vi "上转向轴压装.vi"() -> ()   [LabVIEW 2020]
uses:
  Global_Variable/Global.vi
  Global_Variable/A131258.vi
  Database/Global1.vi
  <vilib>/addons/database/Connection.llb/DB Tools Open Connec (String).vi
  <vilib>/addons/database/Connection.llb/Conn Execute.vi
  <vilib>/addons/database/Recordset.llb/Rec Fetch Recordset Data (R).vi
  <vilib>/addons/database/NI_Database_API.lvlib
panel:
  out "标尺_Event":refnum<user-event>
  out "压装曲线":cluster{dbl[], dbl[]}[](graph)
  out "RESULT":string
  out "PRODUCTID":string
  out "USERID":string
  out "前序deviceID":string
  out "deviceID":string
  out "CODE_ID":string
  in  "判定结果 3":bool[][](array[boolean])=[[TRUE]]
  out "第一段压装位移内波动压力(KN)":dbl format="%_5g"
  out "第二段压装位移内波动压力(KN)":dbl format="%_5g"
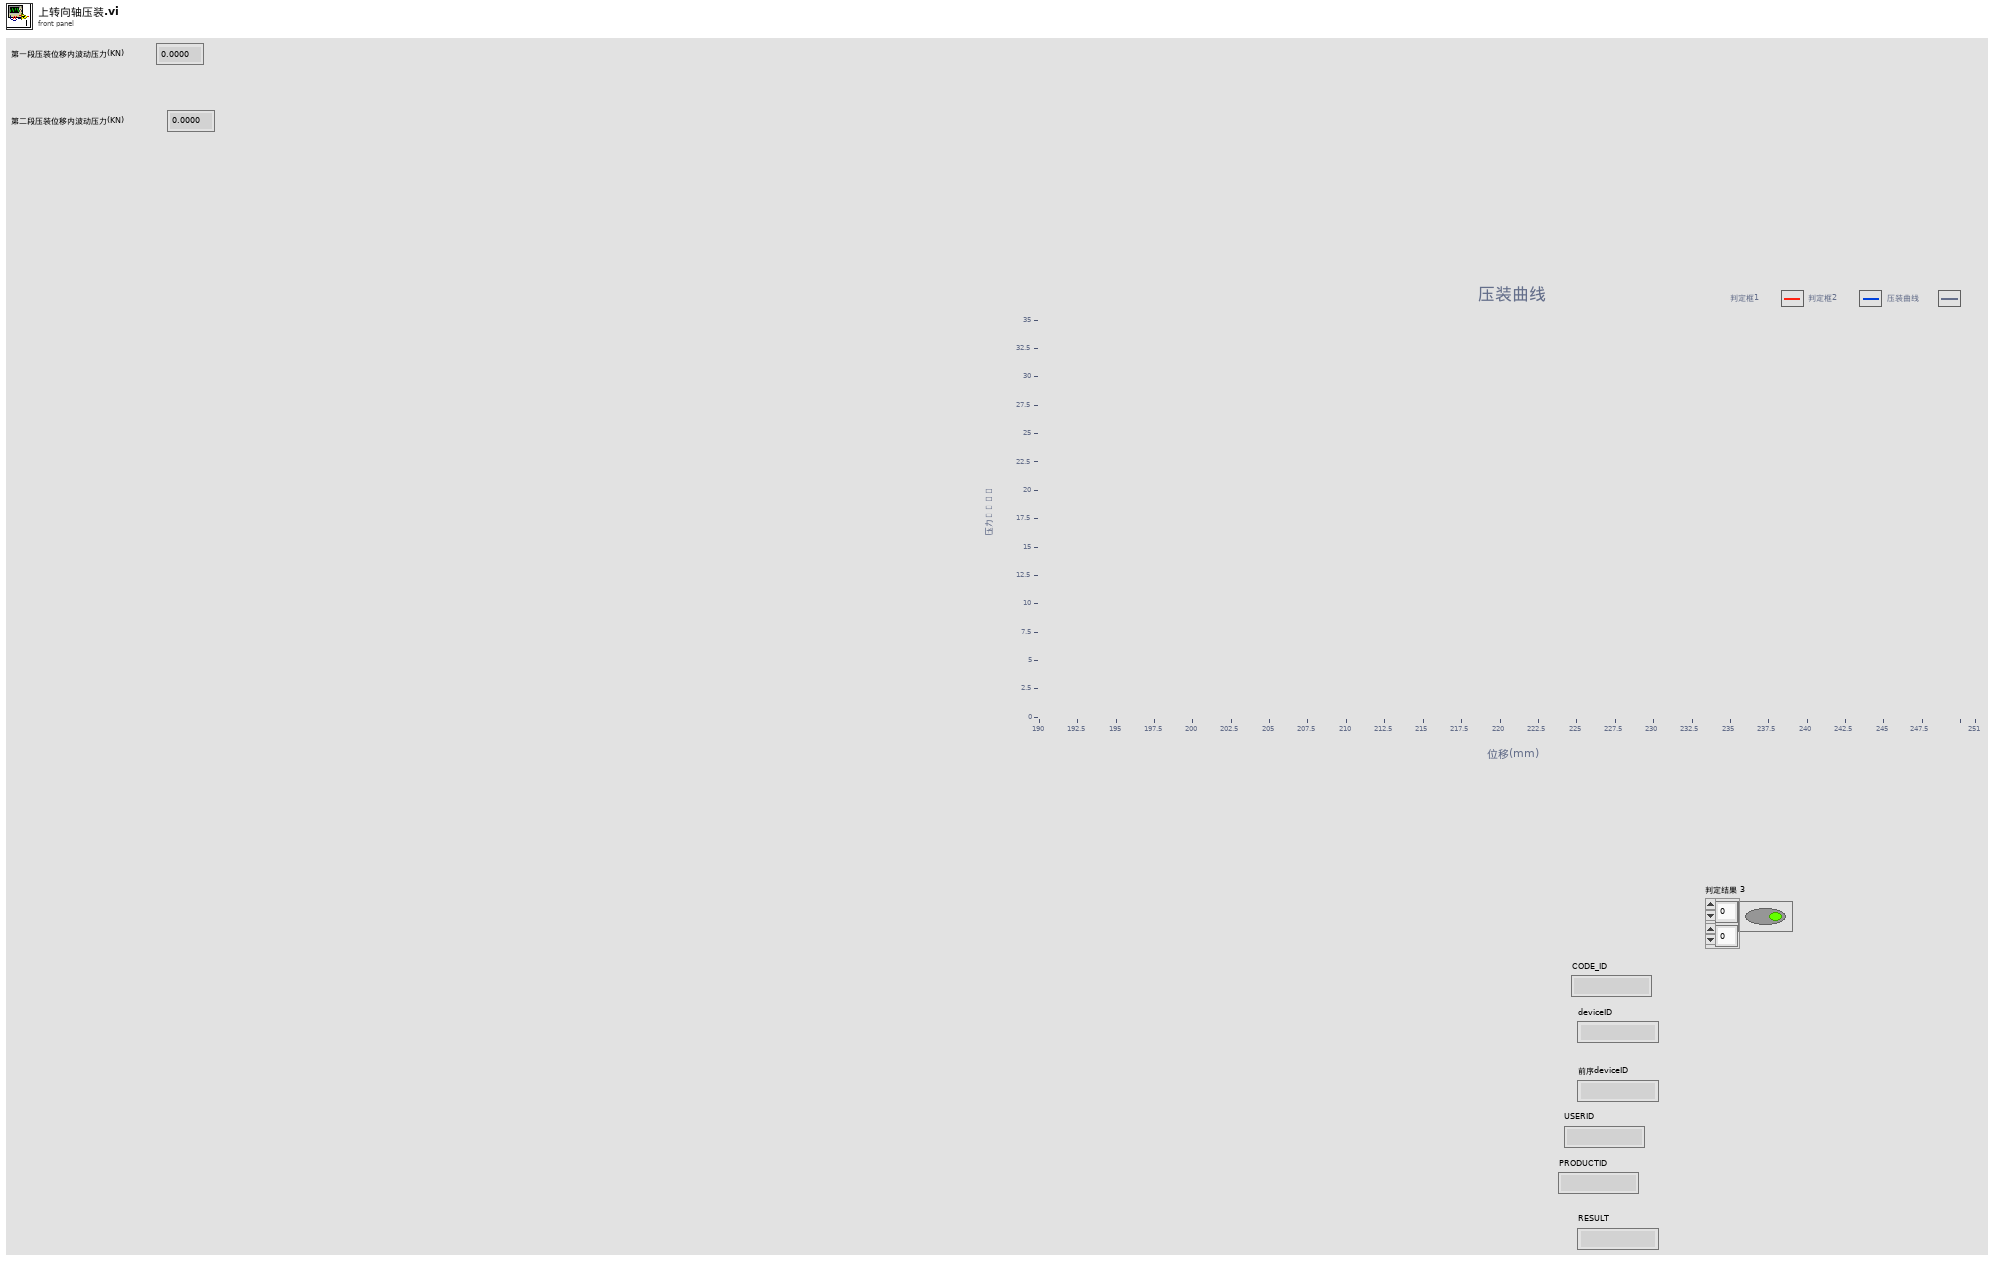
[diagram p1: front panel]
types:
  T1 = cluster{"第一段判定框位移":cluster{"单位":string, "下限":dbl, "上限":dbl}, "第一段判定框压力":cluster{"单位":string, "下限":dbl, "上限":dbl}, "低二段判定框位移":cluster{"单位":string, "下限":dbl, "上限":dbl}, "第二段判定框压力":cluster{"单位":string, "下限":dbl, "上限":dbl}}
  T2 = cluster{"第一段压力最大值":cluster{"单位":string, "下限":dbl, "上限":dbl}, "第一段压力最小值":cluster{"单位":string, "下限":dbl, "上限":dbl}, "压装最终位移":cluster{"单位":string, "下限":dbl, "上限":dbl}}
  T3 = cluster{"第一段压力最大值":cluster{"单位":string, "下限":dbl, "上限":dbl}, "第一段压力最小值":cluster{"单位":string, "下限":dbl, "上限":dbl}, "第二段压力最大值":cluster{"单位":string, "下限":dbl, "上限":dbl}, "第二段压力最小值":cluster{"单位":string, "下限":dbl, "上限":dbl}, "压装最终位移":cluster{"单位":string, "下限":dbl, "上限":dbl}}
  T4 = typedef "NI_Database_API.lvlib/Conn ObjectReference.ctl" = refnum<k1>
  T5 = typedef "NI_Database_API.lvlib/Rec ObjectReference.ctl" = refnum<k1>
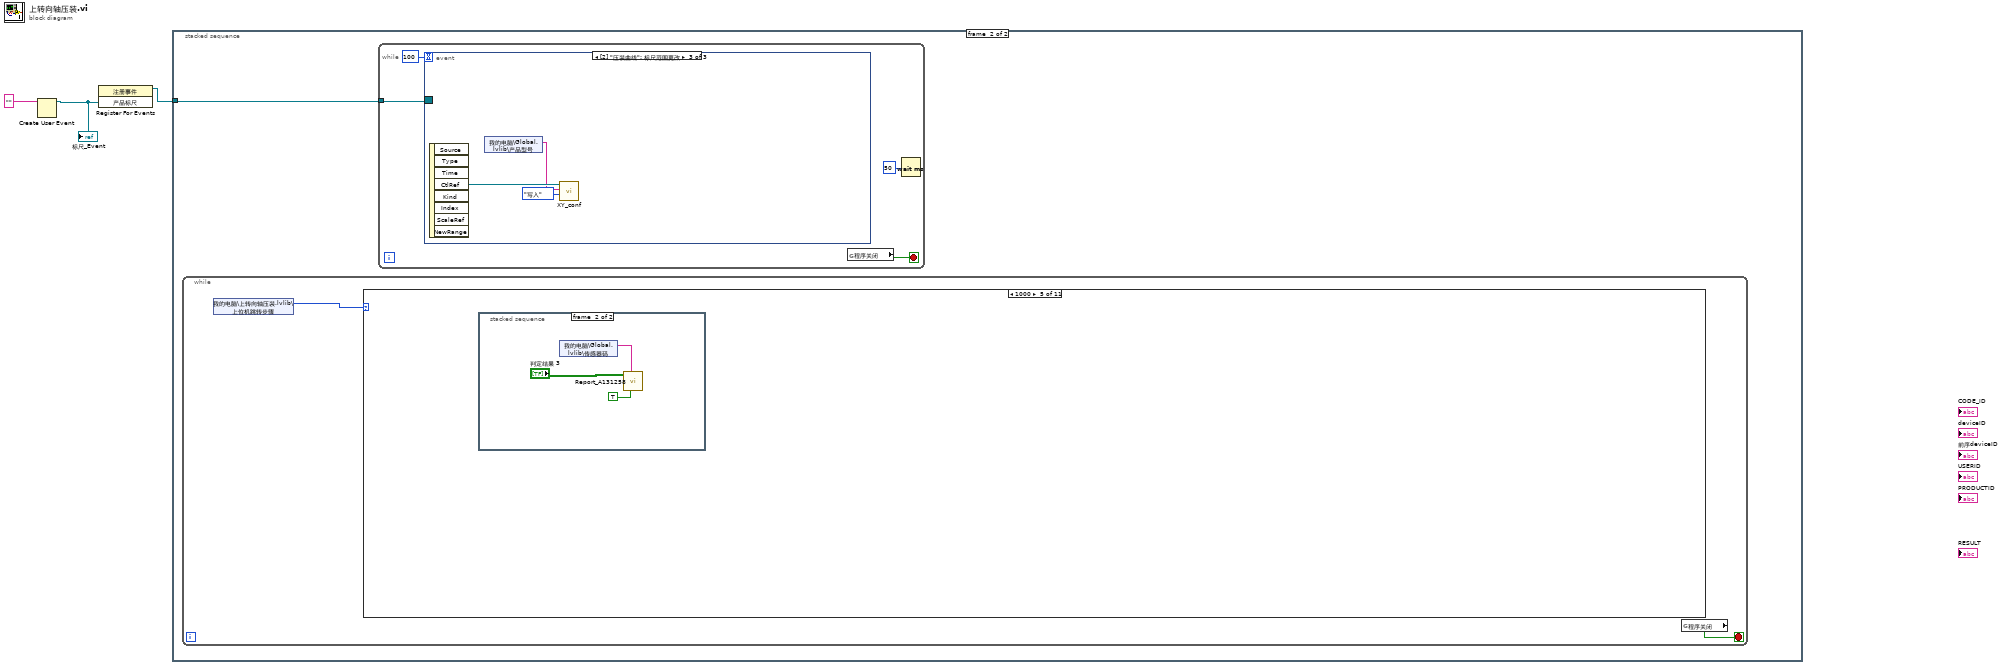
[diagram p0: block diagram]
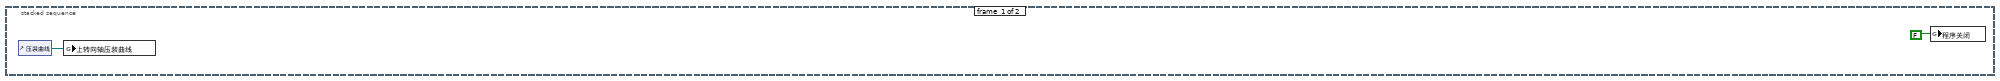
[diagram p2: hidden frame]
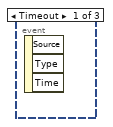
[diagram p3: hidden frame]
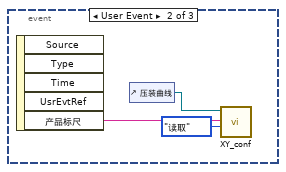
[diagram p4: hidden frame]
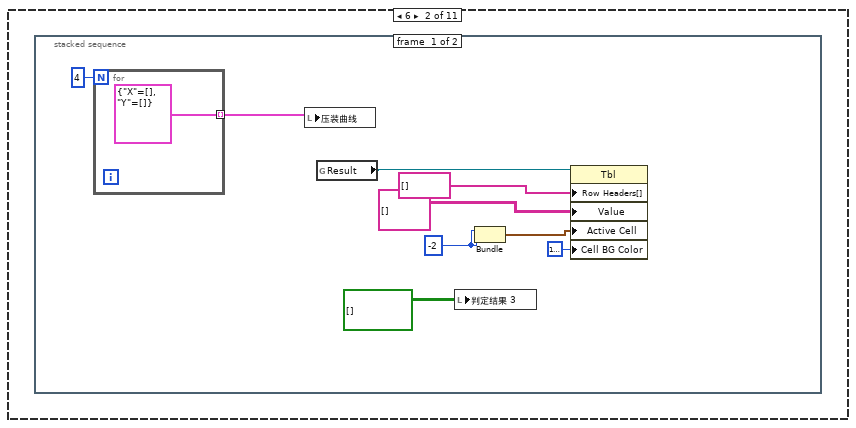
[diagram p6: hidden frame]
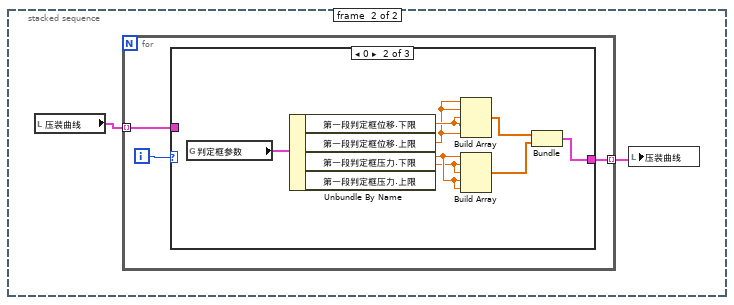
[diagram p7: hidden frame]
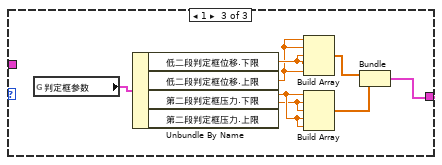
[diagram p9: hidden frame]
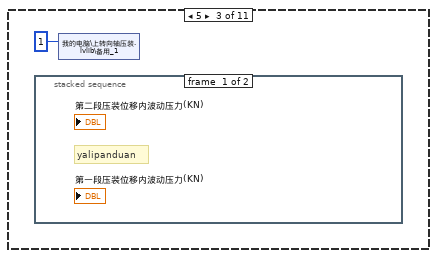
[diagram p10: hidden frame]
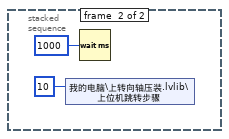
[diagram p11: hidden frame]
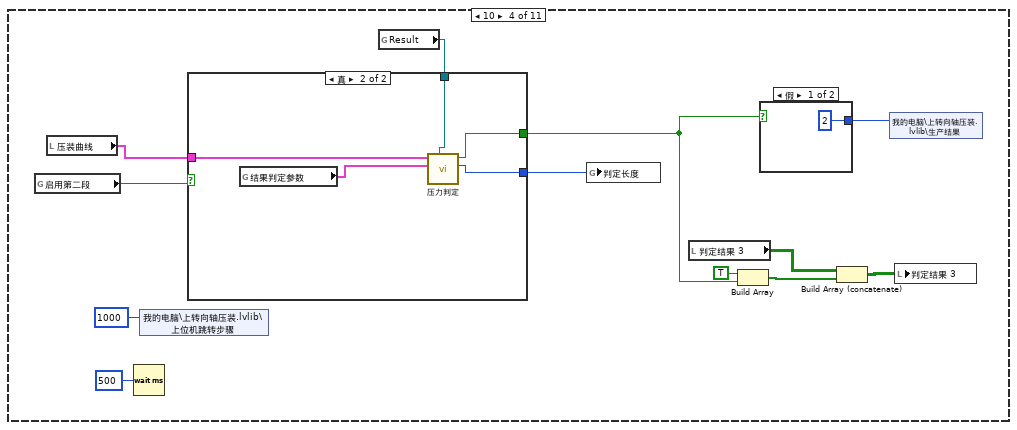
[diagram p12: hidden frame]
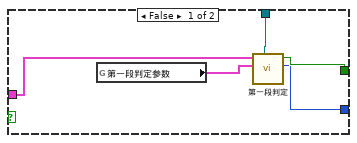
[diagram p13: hidden frame]
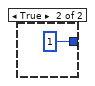
[diagram p14: hidden frame]
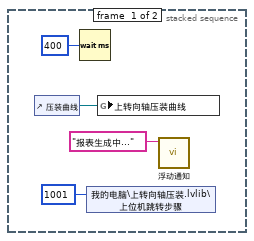
[diagram p15: hidden frame]
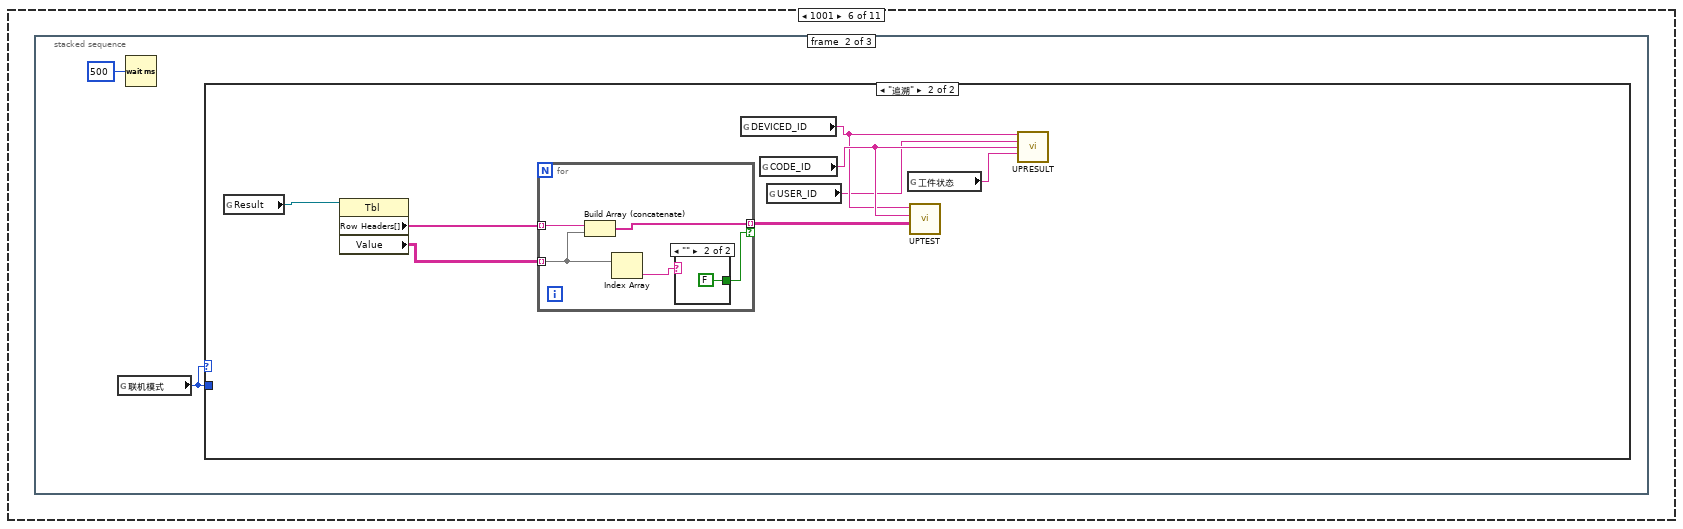
[diagram p16: hidden frame]
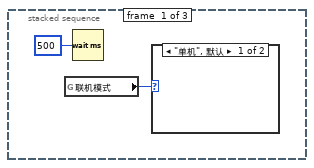
[diagram p17: hidden frame]
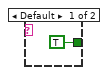
[diagram p20: hidden frame]
diagram:
  n1 = Create User Event(user event datatype="" ("产品标尺")) -> (user event=w2:refnum<user-event>)  [unwired: 1 in, 1 out]
  "标尺_Event" <- w2
  n2 = register-events(w2) -> (reference out=w1:refnum<event-registration>)  [unwired: 2 in, 1 out]
  n3 = stacked-sequence {
    tunnel: w1 -> [_ w6]
    frame #0 {
      n4 = control-ref of="压装曲线"() -> (w4:refnum<vi>)
      n5 = global write "A131258.vi" "上转向轴压装曲线"(w4) -> ()
      n6 = global write "Global.vi" "程序关闭"(FALSE ("程序关闭")) -> ()
    }
    frame #1 {
      n7 = while {
        stop <- w18 stop-if-true
        n8 = shared-variable "我的电脑\\上转向轴压装.lvlib\\上位机跳转步骤"() -> (w17:u16)  [unwired: 1 in, 1 out]
        n9 = case shown="1000" w17 {
          frame 0, Default {
          }
          frame 6 {
            n10 = stacked-sequence {
              frame #0 {
                w22 = -2
                n11 = for {
                  N: 4 -> [_]
                  tunnel: [cluster{"X":dbl[], "Y":dbl[]} {"X"=[], "Y"=[]}] -> w27 mode=indexing
                }
                n12 = local write "压装曲线"(w27) -> ()
                n13 = global read "Global.vi" "Result"() -> (w25:refnum<vi>)
                n14 = local write "判定结果 3"(bool[][] [] ("判定结果 3")) -> ()
                n15 = Bundle(w22, w22) -> (w21:cluster{i32, i32})  [unwired: 1 in]
                n16 = property class="Tbl"(reference=w25, "Row Headers[]"=string[] [] ("行首字符串[]"), "Value"=string[][] [] ("值"), "Active Cell"=w21, "Cell BG Color"=u32 16777216 ("活动单元格:单元格背景色")) -> ()  [unwired: 1 in, 2 out]
              }
              frame #1 {
                n17 = local read "压装曲线"() -> (w30:cluster{dbl[], dbl[]}[])
                n18 = for {
                  tunnel: [w31] -> w29 mode=indexing
                  tunnel: w30 -> [w32] mode=indexing
                  i -> [w33]
                  n19 = case shown="0" w33 {
                    tunnel: [w34 w35 w50] -> w31
                    tunnel: w32 -> [w34 _ _]
                    frame Default {
                    }
                    frame 0 {
                      n20 = global read "Global.vi" "判定框参数"() -> (w36:T1)
                      n21 = Unbundle By Name(w36) -> ("第一段判定框位移.下限"=w40:dbl, "第一段判定框位移.上限"=w39:dbl, "第一段判定框压力.下限"=w38:dbl, "第一段判定框压力.上限"=w37:dbl)
                      n22 = Build Array(w39, w39, w40, w40, w39) -> (w42:dbl[])
                      n23 = Build Array(w38, w37, w37, w38, w38) -> (w41:dbl[])
                      n24 = Bundle(w42, w41) -> (w35:cluster{dbl[], dbl[]})  [unwired: 1 in]
                    }
                    frame 1 {
                      n25 = global read "Global.vi" "判定框参数"() -> (w43:T1)
                      n26 = Unbundle By Name(w43) -> ("低二段判定框位移.下限"=w47:dbl, "低二段判定框位移.上限"=w46:dbl, "第二段判定框压力.下限"=w45:dbl, "第二段判定框压力.上限"=w44:dbl)
                      n27 = Build Array(w46, w46, w47, w47, w46) -> (w49:dbl[])
                      n28 = Build Array(w45, w44, w44, w45, w45) -> (w48:dbl[])
                      n29 = Bundle(w49, w48) -> (w50:cluster{dbl[], dbl[]})  [unwired: 1 in]
                    }
                  }
                }
                n30 = local write "压装曲线"(w29) -> ()
              }
            }
          }
          frame 5 {
            n31 = stacked-sequence {
              frame #0 {
                # "yalipanduan"
              }
              frame #1 {
                n32 = shared-variable "我的电脑\\上转向轴压装.lvlib\\上位机跳转步骤"(u16 10 ("上位机跳转步骤")) -> ()  [unwired: 1 in, 1 out]
                n33 = Wait (ms)(milliseconds to wait=u32 1000 ("等待时间（毫秒）")) -> ()  [unwired: 1 out]
              }
            }
            n34 = shared-variable "我的电脑\\上转向轴压装.lvlib\\备用_1"(u16 1 ("备用_1")) -> ()  [unwired: 1 in, 1 out]
          }
          frame 10 {
            n35 = global read "Global.vi" "启用第二段"() -> (w62:bool)
            n36 = local read "压装曲线"() -> (w61:cluster{dbl[], dbl[]}[])
            n37 = Wait (ms)(milliseconds to wait=u32 500 ("等待时间（毫秒）")) -> ()  [unwired: 1 out]
            n38 = shared-variable "我的电脑\\上转向轴压装.lvlib\\上位机跳转步骤"(u16 1000 ("上位机跳转步骤")) -> ()  [unwired: 1 in, 1 out]
            n39 = global read "Global.vi" "Result"() -> (w60:refnum<vi>)
            n40 = case shown="真" w62 {
              tunnel: w61 -> [w68 w75]
              tunnel: w60 -> [w70 w73]
              tunnel: [w69 w72] -> w58
              tunnel: [w66 w71] -> w59
              frame False {
                n41 = global read "Global.vi" "第一段判定参数"() -> (w67:T2)
                n42 = call "第一段判定.vi"("Result"=w70, "最大值判定"=w67, "XY曲线"=w68) -> ("大小"=w66:i32, "OK？"=w69:bool)  [unwired: 7 in]
              }
              frame True {
                n43 = global read "Global.vi" "结果判定参数"() -> (w74:T3)
                n44 = call "压力判定.vi"("Result"=w73, "判定参数"=w74, "XY曲线"=w75) -> ("大小"=w71:i32, "OK？"=w72:bool)  [unwired: 7 in]
              }
            }
            n45 = global write "Global.vi" "判定长度"(w59) -> ()
            n46 = local read "判定结果 3"() -> (w55:bool[][])
            n47 = Build Array(TRUE ("元素"), w58) -> (w56:bool[])
            n48 = case shown="假" w58 {
              tunnel: [u16 2 ("生产结果") u16 1 ("生产结果")] -> w65
              frame False {
              }
              frame True {
              }
            }
            n49 = Build Array (concatenate)(w55, w56) -> (w54:bool[][])
            n50 = shared-variable "我的电脑\\上转向轴压装.lvlib\\生产结果"(w65) -> ()  [unwired: 1 in, 1 out]
            n51 = local write "判定结果 3"(w54) -> ()
          }
          frame 1000 {
            n52 = stacked-sequence {
              frame #0 {
                n53 = control-ref of="压装曲线"() -> (w78:refnum<vi>)
                n54 = Wait (ms)(milliseconds to wait=u32 400 ("等待时间（毫秒）")) -> ()  [unwired: 1 out]
                n55 = shared-variable "我的电脑\\上转向轴压装.lvlib\\上位机跳转步骤"(u16 1001 ("上位机跳转步骤")) -> ()  [unwired: 1 in, 1 out]
                n56 = global write "A131258.vi" "上转向轴压装曲线"(w78) -> ()
                n57 = call "浮动通知.vi"("通知内容"="报表生成中..." ("Status")) -> ()  [unwired: 11 in]
              }
              frame #1 {
                n58 = shared-variable "我的电脑\\Global.lvlib\\传感器码"() -> (w84:string)  [unwired: 1 in, 1 out]
                n59 = call "Report_A131258.vi"("文件重命名"=TRUE, "文件名称"=w84, "布尔数组"="判定结果 3") -> ()  [unwired: 8 in, 1 out]
              }
            }
          }
          frame 1001 {
            n60 = stacked-sequence {
              frame #0 {
                n61 = global read "Global1.vi" "联机模式"() -> (w86:enum16{"单机", "追溯"})
                n62 = Wait (ms)(milliseconds to wait=u32 500 ("等待时间（毫秒）")) -> ()  [unwired: 1 out]
                n63 = case shown="\"单机\", 默认" w86 {
                  frame "单机", Default {
                  }
                  frame "追溯" {
                  }
                }
              }
              frame #1 {
                n64 = global read "Global1.vi" "联机模式"() -> (w88:enum16{"单机", "追溯"})
                n65 = Wait (ms)(milliseconds to wait=u32 500 ("毫秒计时值")) -> ()  [unwired: 1 out]
                n66 = case shown="\"追溯\"" w88 {
                  tunnel: w88 -> [_ _]
                  frame "单机", Default {
                  }
                  frame "追溯" {
                    n67 = global read "Global.vi" "Result"() -> (w96:refnum<vi>)
                    n68 = property class="Tbl"(reference=w96) -> ("Row Headers[]"=w95:string[], "Value"=w94:string[][])  [unwired: 1 in, 2 out]
                    n69 = for {
                      tunnel: w95 -> [w101] mode=indexing
                      tunnel: w94 -> [w99] mode=indexing
                      tunnel: [w100] -> w93 mode=indexing if=w97
                      n70 = Build Array (concatenate)(w101, w99) -> (w100:string[])
                      n71 = Index Array(array=w99) -> (element=w98:string)  [unwired: 1 in]
                      n72 = case shown="\"\"" w98 {
                        tunnel: [TRUE FALSE] -> w97
                        frame Default {
                        }
                        frame "" {
                        }
                      }
                    }
                    n73 = global read "Global.vi" "DEVICED_ID"() -> (w91:string)
                    n74 = global read "Global.vi" "CODE_ID"() -> (w92:string)
                    n75 = global read "Global.vi" "USER_ID"() -> (w90:string)
                    n76 = global read "追溯全部变量.vi" "工件状态"() -> (w89:string)
                    n77 = call "UPTEST.vi"("Result"=w93, "CODE_ID"=w92, "DEVICE_ID"=w91) -> ()  [unwired: 6 in, 1 out]
                    n78 = call "UPRESULT.vi"("DEVICE_ID"=w91, "USER_ID"=w90, "CODE_ID"=w92, "RESULT_VALUE"=w89) -> ()  [unwired: 11 in, 1 out]
                  }
                }
              }
              frame #2 {
                n79 = shared-variable "我的电脑\\上转向轴压装.lvlib\\备用_1"(u16 0 ("备用_1")) -> ()  [unwired: 1 in, 1 out]
                n80 = shared-variable "我的电脑\\上转向轴压装.lvlib\\上位机跳转步骤"(u16 0 ("上位机跳转步骤")) -> ()  [unwired: 1 in, 1 out]
              }
            }
          }
          frame 2000 {
            n81 = stacked-sequence {
              frame #0 {
                n82 = shared-variable "我的电脑\\Global.lvlib\\传感器码"("" ("传感器码")) -> ()  [unwired: 1 in, 1 out]
                n83 = Wait (ms)(milliseconds to wait=u32 200 ("等待时间（毫秒）")) -> ()  [unwired: 1 out]
                n84 = shared-variable "我的电脑\\上转向轴压装.lvlib\\上位机跳转步骤"(u16 2005 ("备用1")) -> ()  [unwired: 1 in, 1 out]
              }
              frame #1 {
                (unwired) cluster{u32, u32}[] [{12369084, 12369084}, {11776947, 11776947}, {11776947, 11776947}, {12369084, 12369084}]
                w110 = "请扫码！" ("通知内容")
                n85 = call "浮动通知.vi"("通知内容"=w110) -> ()  [unwired: 11 in]
                n86 = call "输入框.vi"("提示信息"=w110) -> ("条形码输出"=w109:string)
                n87 = shared-variable "我的电脑\\Global.lvlib\\传感器码"(w109) -> ()  [unwired: 1 in, 1 out]
              }
            }
          }
          frame 2001 {
            n88 = global read "Global1.vi" "联机模式"() -> (w111:enum16{"单机", "追溯"})
            n89 = case shown="\"追溯\"" w111 {
              frame "单机", Default {
                n90 = shared-variable "我的电脑\\上转向轴压装.lvlib\\上位机跳转步骤"(u16 2002 ("备用1")) -> ()  [unwired: 1 in, 1 out]
              }
              frame "追溯" {
                n91 = global read "Global.vi" "FRE_ID"() -> (w114:string)
                n92 = Equal?(x=w114, y="") -> (x = y?=w115:bool)
                n93 = case shown="真" w115 {
                  frame False {
                    n94 = stacked-sequence {
                      frame #0 {
                        n95 = shared-variable "我的电脑\\Global.lvlib\\传感器码"() -> (w118:string)  [unwired: 1 in, 1 out]
                        n96 = call "Get_CODE_ID.vi"("CODE_SENSOR"=w118) -> ("CODE_ID"=w117:string)  [unwired: 10 in]
                        n97 = global write "Global.vi" "CODE_ID"(w117) -> ()
                        n98 = Wait (ms)(milliseconds to wait=u32 50 ("等待时间（毫秒）")) -> ()  [unwired: 1 out]
                      }
                      frame #1 {
                        n99 = global read "Global.vi" "FRE_ID"() -> (w120:string)
                        n100 = global read "Global.vi" "CODE_ID"() -> (w119:string)
                        n101 = global read "Global1.vi" "联机模式"() -> (w140:enum16{"单机", "追溯"})
                        n102 = call "GetSQLstring.vi"("联机模式"=w140) -> ("错误输出"=w138:errorcluster, "连接字符串"=w139:string)  [unwired: 9 in]
                        n103 = Concatenate Strings("SELECT RESULT_VALUE FROM RESULT  WHERE DEVICE_ID = \n" ("table"), w120, " AND CODE_ID=" ("字符串"), w119) -> (w137:string)
                        n104 = call-poly <vilib>:"DB Tools Open Connection.vi"("error in (no error)"=w138, "connection information"=w139) -> ("error out"=w131:errorcluster, "connection reference"=w132:T4)  [unwired: 6 in]
                        n105 = call-poly <vilib>:"DB Tools Execute Query.vi"("error in (no error)"=w131, "SQL query"=w137, "connection reference"=w132) -> ("error out"=w135:errorcluster, "recordset reference"=w136:T5)  [unwired: 5 in]
                        n106 = call-poly <vilib>:"DB Tools Fetch Recordset Data.vi"("error in (no error)"=w135, "recordset reference"=w136) -> ("error out"=w129:errorcluster, "recordset data"=w134:variant[][])  [unwired: 3 in, 1 out]
                        n107 = Variant To Data(error in=w129, type=string[][] [], Variant=w134) -> (data=w125:string[][], error out=w123:errorcluster)
                        n108 = call <vilib>:"Clear Errors.vi"("error in (no error)"=w123) -> ("error out"=w122:errorcluster)  [unwired: 5 in, 1 out]
                        n109 = Index Array(array=w125, index (row)=0 ("索引 (行)")) -> (element=w127:string[])  [unwired: 1 in]
                        n110 = call <vilib>:"Simple Error Handler.vi"("error in (no error)"=w122) -> ()  [unwired: 4 in, 5 out]
                        n111 = Index Array(array=w127, index=0 ("索引 (行)")) -> (element=w124:string)
                        n112 = case shown="\"OK\"" w124 {
                          frame "假", Default {
                          }
                          frame "" {
                            n113 = global read "Global.vi" "上序状态"() -> (w143:refnum<vi>)
                            n114 = shared-variable "我的电脑\\上转向轴压装.lvlib\\上位机跳转步骤"(u16 5000 ("备用1")) -> ()  [unwired: 1 in, 1 out]
                            n115 = property class="Str"(reference=w143, "Text.Text"="漏序" ("上序状态显示"), "Text.BGColor"=u32 16776960 ("文本.文本颜色:背景色")) -> ()  [unwired: 1 in, 2 out]
                          }
                          frame "OK" {
                            n116 = global read "Global.vi" "上序状态"() -> (w147:refnum<vi>)
                            n117 = shared-variable "我的电脑\\Global.lvlib\\传感器码"() -> (w150:string)  [unwired: 1 in, 1 out]
                            n118 = property class="Str"(reference=w147, "Text.Text"="合格" ("上序状态显示"), "Text.BGColor"=u32 6618880 ("文本.文本颜色:背景色")) -> ()  [unwired: 1 in, 2 out]
                            n119 = String Length(string=w150) -> (length=w151:i32)
                            n120 = Greater?(x=w151, y=4) -> (0:w148:bool)
                            n121 = case shown="真" w148 {
                              frame False {
                              }
                              frame True {
                                n122 = shared-variable "我的电脑\\上转向轴压装.lvlib\\上位机跳转步骤"(u16 2002 ("备用1")) -> ()  [unwired: 1 in, 1 out]
                              }
                            }
                          }
                          frame "NG" {
                            n123 = global read "Global.vi" "上序状态"() -> (w155:refnum<vi>)
                            n124 = shared-variable "我的电脑\\上转向轴压装.lvlib\\上位机跳转步骤"(u16 5000 ("备用1")) -> ()  [unwired: 1 in, 1 out]
                            n125 = property class="Str"(reference=w155, "Text.Text"="不合格" ("上序状态显示"), "Text.BGColor"=u32 16711680 ("文本.文本颜色:背景色")) -> ()  [unwired: 1 in, 2 out]
                          }
                        }
                      }
                    }
                  }
                  frame True {
                    n126 = flat-sequence {
                      frame #0 {
                        n127 = global read "Global.vi" "上序状态"() -> (w159:refnum<vi>)
                        n128 = property class="Str"(reference=w159, "Text.Text"="首序" ("上序状态显示"), "Text.BGColor"=u32 6618880 ("文本.文本颜色:背景色")) -> ()  [unwired: 1 in, 2 out]
                      }
                      frame #1 {
                        n129 = global read "Global.vi" "PRODUCT_ID"() -> (w161:string)
                        n130 = shared-variable "我的电脑\\Global.lvlib\\传感器码"() -> (w162:string)  [unwired: 1 in, 1 out]
                        n131 = Wait (ms)(milliseconds to wait=u32 50 ("等待时间（毫秒）")) -> ()  [unwired: 1 out]
                        n132 = call "INSERT_CODE.vi"("PRODUCT_ID"=w161, "CODE_SENSOR"=w162) -> ()  [unwired: 7 in, 1 out]
                      }
                      frame #2 {
                        n133 = shared-variable "我的电脑\\Global.lvlib\\传感器码"() -> (w165:string)  [unwired: 1 in, 1 out]
                        n134 = String Length(string=w165) -> (length=w164:i32)
                        n135 = Greater?(x=w164, y=4) -> (0:w166:bool)
                        n136 = case shown="真" w166 {
                          frame False {
                          }
                          frame True {
                            n137 = shared-variable "我的电脑\\上转向轴压装.lvlib\\上位机跳转步骤"(u16 2002 ("备用1")) -> ()  [unwired: 1 in, 1 out]
                          }
                        }
                      }
                    }
                  }
                }
              }
            }
          }
          frame 2005 {
            n138 = shared-variable "我的电脑\\Global.lvlib\\传感器码"() -> (w170:string)  [unwired: 1 in, 1 out]
            n139 = String Length(string=w170) -> (length=w171:i32)
            n140 = Greater?(x=w171, y=4) -> (0:w168:bool)
            n141 = case shown="真" w168 {
              frame False {
              }
              frame True {
                n142 = shared-variable "我的电脑\\上转向轴压装.lvlib\\上位机跳转步骤"(u16 2001 ("备用1")) -> ()  [unwired: 1 in, 1 out]
              }
            }
          }
          frame 2 {
            (unwired) cluster{u32, u32}[] [{12369084, 12369084}, {11776947, 11776947}, {11776947, 11776947}, {12369084, 12369084}]
            (unwired) u32 12369084
            n143 = shared-variable "我的电脑\\上转向轴压装.lvlib\\生产结果"(u16 0 ("生产结果")) -> ()  [unwired: 1 in, 1 out]
            n144 = for {
              N: 4 -> [_]
              tunnel: [cluster{"X":dbl[], "Y":dbl[]} {"X"=[], "Y"=[]}] -> w173 mode=indexing
            }
            n145 = local write "压装曲线"(w173) -> ()
          }
          frame 7 {
            n146 = local read "压装曲线"() -> (w177:cluster{dbl[], dbl[]}[])
            n147 = for {
              tunnel: [w181] -> w178 mode=indexing
              tunnel: w177 -> [w180] mode=indexing
              i -> [w179]
              n148 = case shown="2" w179 {
                tunnel: [w182 w188] -> w181
                tunnel: w180 -> [w182 w187]
                frame Default {
                }
                frame 2 {
                  n149 = Unbundle(w187) -> (w192:dbl[], w191:dbl[])
                  n150 = shared-variable "我的电脑\\上转向轴压装.lvlib\\电缸压装参数"() -> (w183:sgl[])  [unwired: 1 in, 1 out]
                  n151 = shared-variable "我的电脑\\上转向轴压装.lvlib\\电缸压装参数"() -> (w184:sgl[])  [unwired: 1 in, 1 out]
                  n152 = Index Array(array=w183, index=1) -> (element=w185:sgl)
                  n153 = Index Array(array=w184, index=0) -> (element=w186:sgl)
                  n154 = Build Array (concatenate)(w192, w185) -> (w190:dbl[])
                  n155 = Build Array (concatenate)(w191, w186) -> (w189:dbl[])
                  n156 = Bundle(w190, w189) -> (w188:cluster{dbl[], dbl[]})  [unwired: 1 in]
                }
              }
            }
            n157 = local write "压装曲线"(w178) -> ()
          }
        }
        n158 = global read "Global.vi" "程序关闭"() -> (w18:bool)
      }
      n159 = while {
        tunnel: w6 -> [w7]
        stop <- w10 stop-if-true
        n160 = event shown="[2] \"压装曲线\": 标尺范围更改" {
          selector: w7 -> [_ _ _]
          dyn-events: _ -> [_ _ _]
          timeout: 100 -> [_ _ _]
          event Timeout {
            n161 = event-data() -> ()  [unwired: 1 in, 3 out]
          }
          event User Event {
            n162 = event-data() -> ("产品标尺"=w13:string)  [unwired: 1 in, 4 out]
            n163 = control-ref of="压装曲线"() -> (w12:refnum<vi>)
            n164 = call "XY_conf.vi"("方式"=enum16{"写入", "读取"}."读取", "产品型号"=w13, "XY图引用"=w12) -> ()  [unwired: 3 in, 1 out]
          }
          event "压装曲线": Scale Range Change {
            n165 = event-data() -> ("CtlRef"=w16:refnum<vi>)  [unwired: 1 in, 7 out]
            n166 = shared-variable "我的电脑\\Global.lvlib\\产品型号"() -> (w15:string)  [unwired: 1 in, 1 out]
            n167 = call "XY_conf.vi"("方式"=enum16{"写入", "读取"}."写入", "产品型号"=w15, "XY图引用"=w16) -> ()  [unwired: 3 in, 1 out]
          }
        }
        n168 = global read "Global.vi" "程序关闭"() -> (w10:bool)
        n169 = Wait (ms)(milliseconds to wait=u32 50 ("等待时间（毫秒）")) -> ()  [unwired: 1 out]
      }
    }
  }
